vi "Client - SEND - Message.vi"(7 "Destination":T1, 8 "error in":errorcluster) -> (0 "error out":errorcluster)   [LabVIEW 2023, in "Client.lvlib" / "Client.lvclass"]
uses:
  Client.lvclass
  Parent/Parent_Class.lvclass
  Child_1/Child_1_Class.lvclass
  Console/Child_1/Child_2_Class.lvclass
  Interface_Class/Interface_Class.lvclass
  Message_Distributor/Parent_Class Messages/Parent -  SEND - Triggered Event Msg/Parent -  SEND - Triggered Event Msg.lvclass
  Client - Ctrl - FGV - Action.ctl
  SW_Interface/Child_3_Class.lvclass
  C:/Users/rodri/LabVIEW_Labs/LabVIEW_GitHub/LV-AF-Project/AF_Architecture/Abstraction_Interface_Class/Abstraction_Interface_Class.lvclass
  C:/Program Files (x86)/National Instruments/LabVIEW 2023/vi.lib/ActorFramework/Actor/Actor.lvclass
  C:/Users/rodri/LabVIEW_Labs/LabVIEW_GitHub/LV-AF-Project/AF_Architecture/SW_Interface/Child_3_Class.lvclass
  Client - Ctrl - Actor - Destination.ctl
panel:
  in  "Value":string
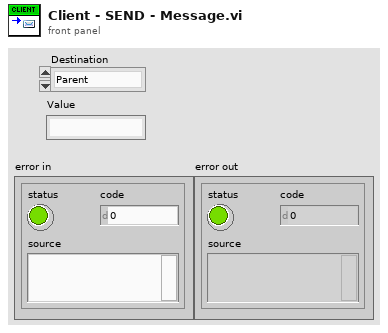
[diagram p1: front panel]
types:
  T1 = typedef "Client.lvlib/Client.lvclass/Client - Ctrl - Actor - Destination.ctl" = enum16{"Parent", "Child_1", "Child_2", "Child_3"}
  T2 = typedef "Client.lvlib/Client.lvclass/Client - Ctrl - FGV - Action.ctl" = enum16{"Int", "Get"}
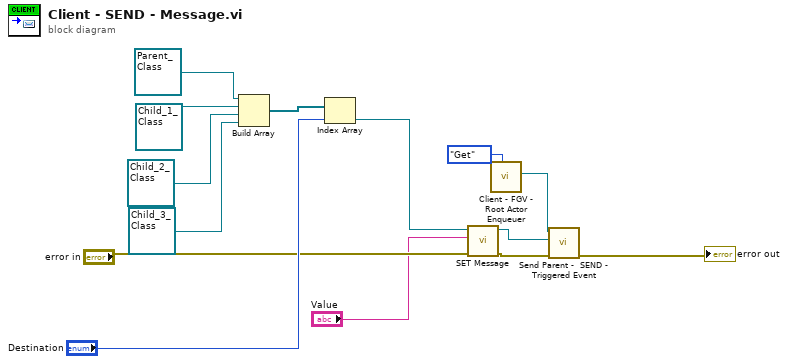
[diagram p0: block diagram]
diagram:
  n1 = Build Array(refnum<class "Parent_Class.lvclass"> refnum ("Actor_Parent.lvlib:Parent_Class.lvclass"), refnum<class "Child_1_Class.lvclass"> refnum ("Actor_Child_1.lvlib:Child_1_Class.lvclass"), refnum<class "Child_2_Class.lvclass"> refnum ("Actor_Child_2.lvlib:Child_2_Class.lvclass"), refnum<class "Child_3_Class.lvclass"> refnum ("Actor_Child_3.lvlib:Child_3_Class.lvclass")) -> (w11:refnum<class>[])
  n2 = Index Array(array=w11, index="Destination") -> (element=w8:refnum<class>)
  n3 = call-dynamic "SET Message.vi"("error in (no error)"="error in", "Data"="Value", "Interface_Class in"=w8) -> ("error out"=w6:errorcluster, "Interface_Class out"=w5:refnum<class "Interface_Class.lvclass">)  [unwired: 7 in]
  n4 = call "Client - FGV - Root Actor Enqueuer.vi"("Action"=Client_-_Ctrl_-_FGV_-_Action."Get") -> ("Root Enqueuer"=w3:refnum<class "Message Enqueuer.lvclass">)  [unwired: 9 in, 1 out]
  n5 = call "Send Parent -  SEND - Triggered Event.vi"("error in (no error)"=w6, "Actor_Interface.lvlib:Interface_Class.lvclass"=w5, "Message Enqueuer"=w3) -> ("error out"=→"error out":errorcluster)  [unwired: 7 in, 1 out]
